vi "Create Device GUI.vi"(8 "Error In":errorcluster, 9 "Device":i32, 10 "Platform":i32, 11 "Skip Configuration":bool) -> (0 "error constant":errorcluster, 3 "Device Reference":T1)   [LabVIEW 2012]
doc: "A GUI that shows which OpenCL Platforms and Devices are available. Selecting a platform will populate the devices available for that platform. Once a device is selected, a context can be created by clicking continue.\n\nThe GUI can be bypassed by wiring <b>Skip Configuration</b> to true and providing a Platform and Device number. This is only recommended after running the GUI and becoming familiar with devices and platforms."
uses:
  Non-User VIs/Controls/Device ID.ctl
  Non-User VIs/Buffers/Buffer_states.ctl
  Non-User VIs/Error Checking/Add Error Functional Global.vi
  OpenCLV x64.lvlib
panel:
  in  "Cancel Button":bool
  in  "Continue":bool caption="Create Device"
  out "Device Properties":string[](tree)
  in  "Devices":i32(listbox)
  out "Platform Properties":string[](tree)=["FULL_PROFILE"]
  in  "Platform Names":i32(listbox)
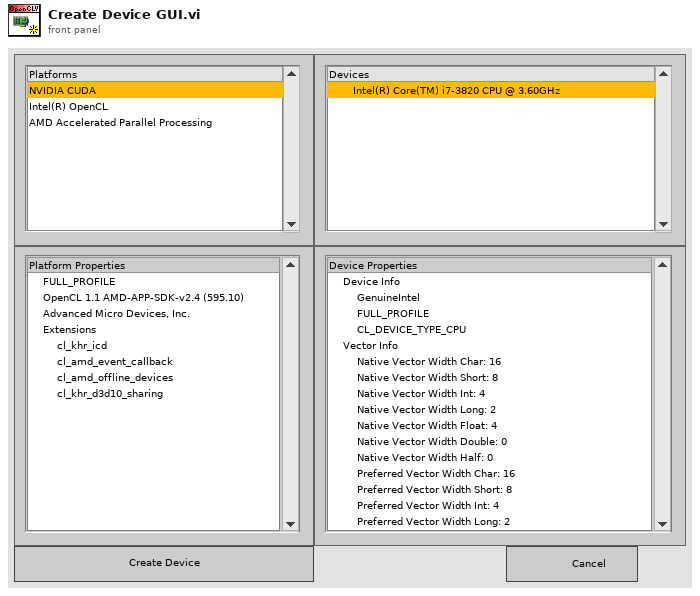
[diagram p1: front panel]
types:
  T1 = typedef "OpenCLV x64.lvlib/Device ID.ctl" = u64
  T2 = typedef "OpenCLV x64.lvlib/Buffer_states.ctl" = enum16{"Purge", "Remove", "Add"}
  T3 = enum8{"Enabled", "Disabled", "Disabled and Grayed Out"}
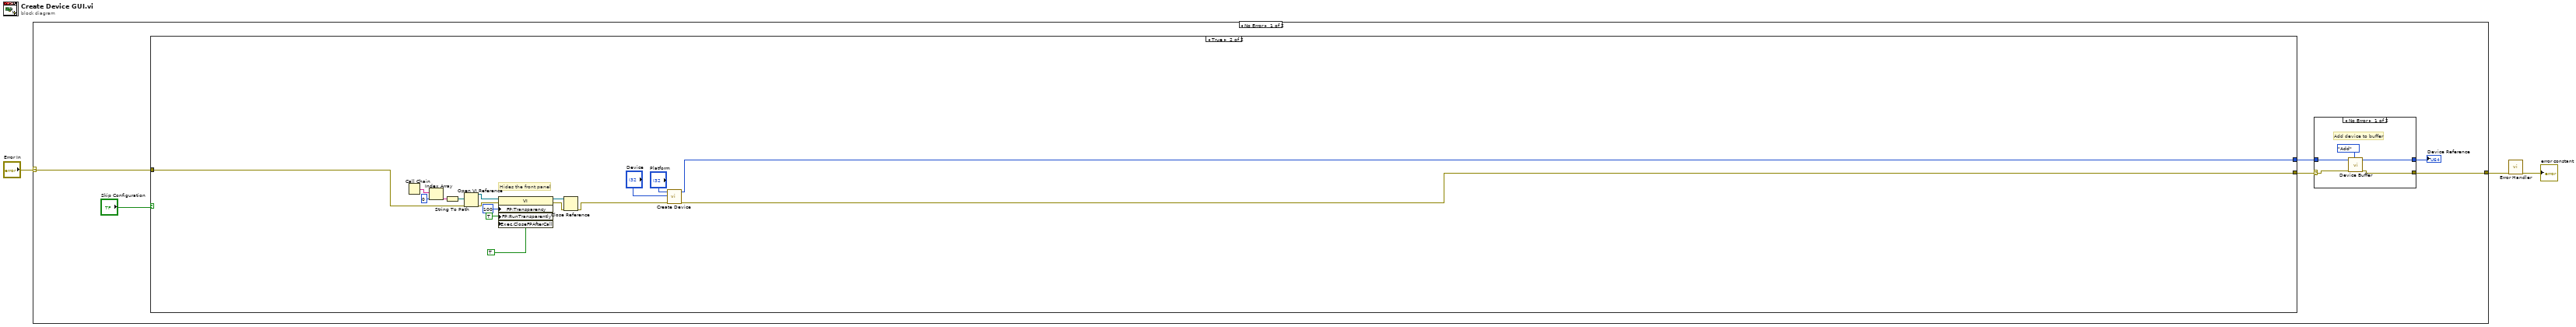
[diagram p0: block diagram]
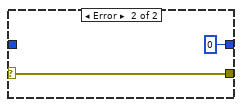
[diagram p2: hidden frame]
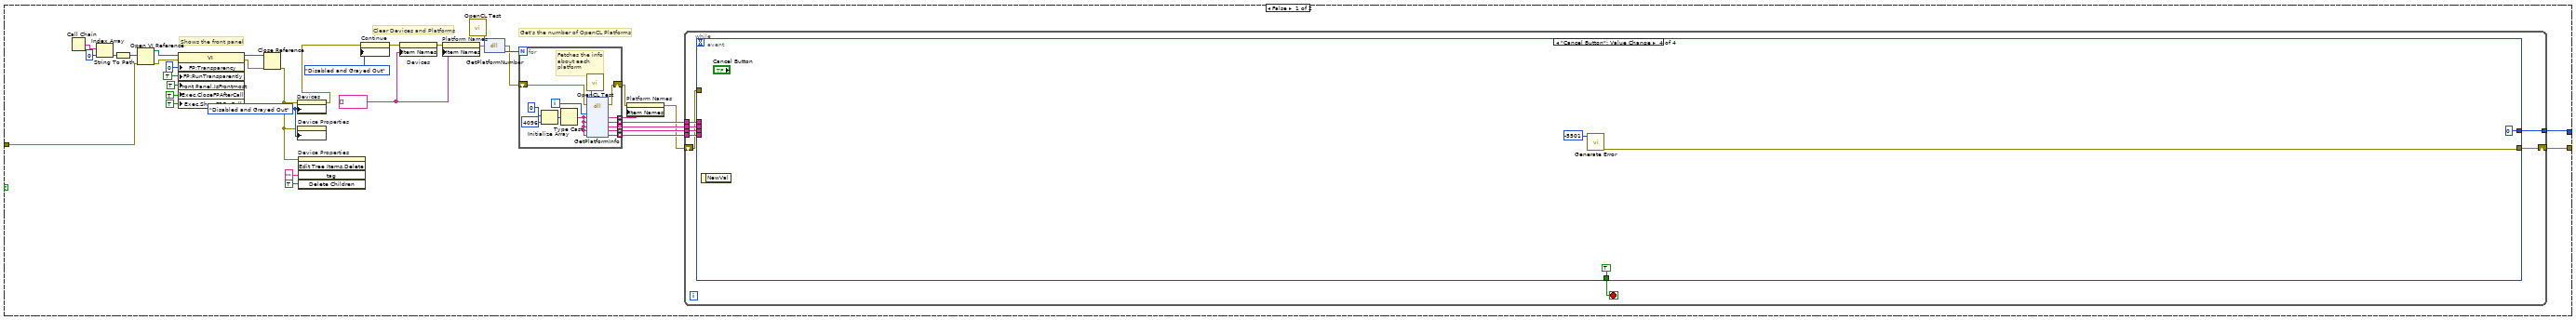
[diagram p3: hidden frame]
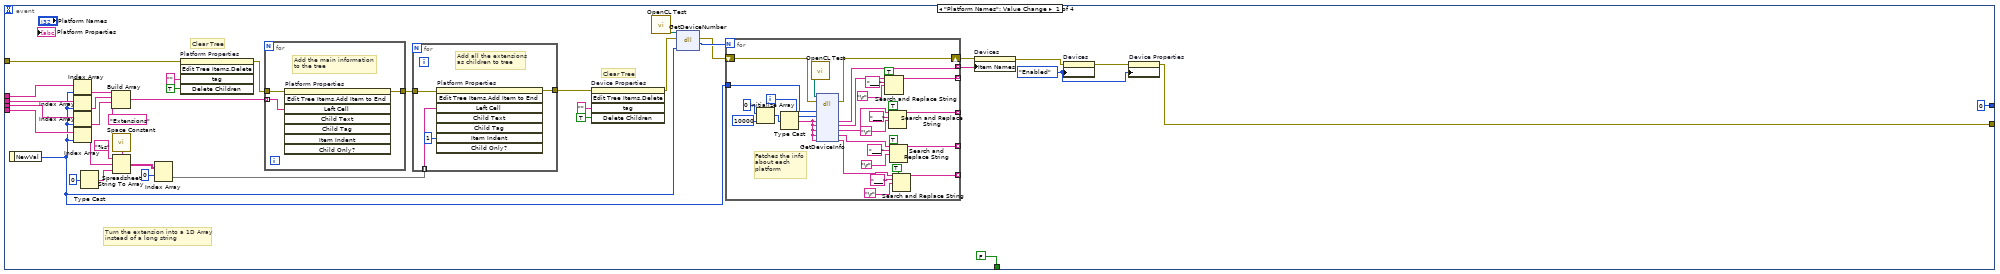
[diagram p4: hidden frame]
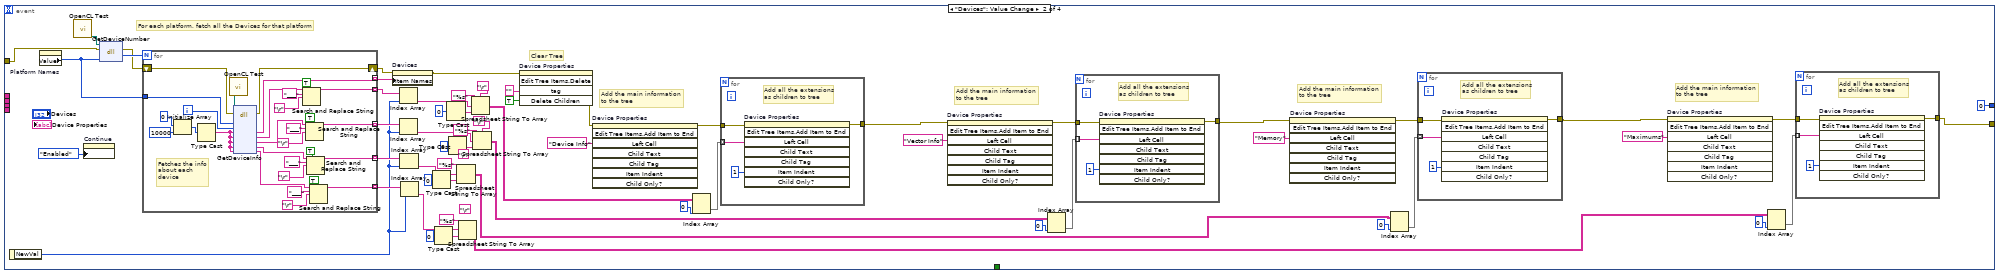
[diagram p5: hidden frame]
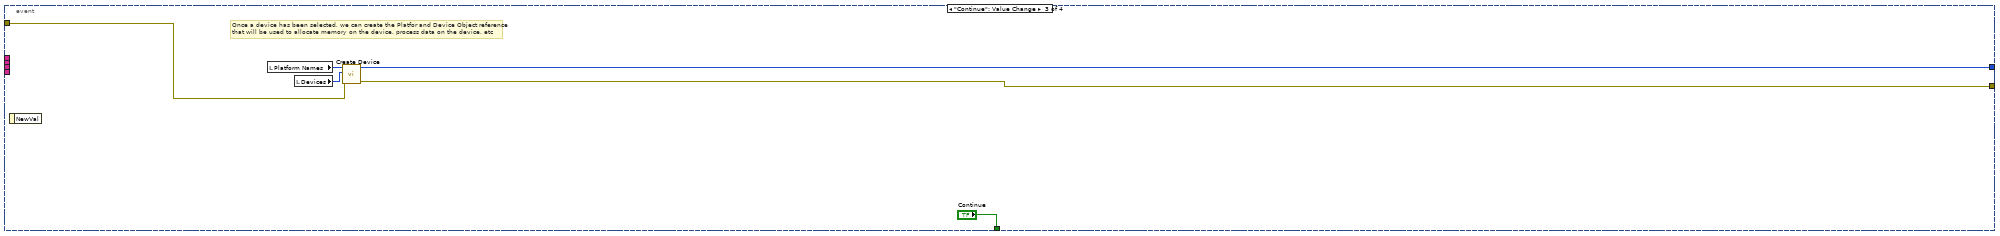
[diagram p6: hidden frame]
diagram:
  n1 = case shown="No Error" "Error In" {
    selector: "Error In" -> [w4 w282]
    tunnel: [w5 w282] -> w2
    frame No Error {
      n2 = case shown="True" "Skip Configuration" {
        tunnel: [w20 w280] -> w7
        tunnel: [w29 w269] -> w8
        tunnel: w4 -> [w17 w265]
        frame False {
          w25 = T3."Disabled and Grayed Out" ("Disabled")
          w43 = string[] [] ("Item Names")
          # "Shows the front panel"
          # "Clear Devices and Platforms"
          # "Get's the number of OpenCL Platforms"
          n3 = Call Chain() -> (call chain=w40:string[])
          n4 = Index Array(array=w40, index=0) -> (element=w38:string)
          n5 = String To Path(string=w38) -> (path=w37:path)
          n6 = Open VI Reference(vi path=w37, error in (no error)=w17) -> (vi reference=w36:refnum<vi>, error out=w35:errorcluster)  [unwired: 4 in]
          n7 = property class="VI"(reference=w36, error in=w35, "FP:Transparency"=u8 0 ("Front Panel Window:Transparency"), "FP:RunTransparently"=TRUE ("Front Panel Window:Run VI Transparently"), "Front Panel.IsFrontmost"=TRUE ("Front Panel Window:Is Frontmost"), "Exec.CloseFPAfterCall"=TRUE ("Execution:Close After Call"), "Exec.ShowFPOnCall"=TRUE ("Execution:Show Front Panel On Call")) -> (reference out=w28:refnum<vi>, error out=w27:errorcluster)
          n8 = Close Reference(reference=w28, error in (no error)=w27) -> (error out=w22:errorcluster)
          n9 = property on="Devices" class="LstBox (strict)"(error in=w22, "DisabledEnum"=w25) -> (error out=w26:errorcluster)  [unwired: 1 in, 1 out]
          n10 = property on="Device Properties" class="Tree (strict)"(error in=w22, "DisabledEnum"=w25) -> ()  [unwired: 1 in, 2 out]
          n11 = invoke on="Device Properties" class="Tree (strict)" method="Edit Tree Items.Delete"(error in=w22, "tag"="" ("Tag"), "Delete Children"=TRUE ("Delete Children?")) -> ()  [unwired: 2 in, 5 out]
          n12 = property on="Continue" class="Bool"(error in=w26, "DisabledEnum"=T3."Disabled and Grayed Out" ("Disabled")) -> (error out=w41:errorcluster)  [unwired: 1 in, 1 out]
          n13 = property on="Devices" class="LstBox (strict)"(error in=w41, "Item Names"=w43) -> (error out=w44:errorcluster)  [unwired: 1 in, 1 out]
          n14 = property on="Platform Names" class="LstBox (strict)"(error in=w44, "Item Names"=w43) -> (error out=w45:errorcluster)  [unwired: 1 in, 1 out]
          n15 = call "OpenCL Test.vi"() -> ("DLL To Use"=w21:path)  [unwired: 11 in]
          n16 = dll-call lib="C:/Users/bme-amcelroy-la/Desktop/OpenCLV/trunk/OpenCLV_x64_1.0/OpenCLV_x64.dll" fn="GetPlatformNumber"(path in=w21, error in=w45) -> (error out=w19:errorcluster, "Number of Platforms"=w47:i32)  [unwired: 1 in, 1 out]
          n17 = for {
            N: w47 -> [_]
            tunnel: [w264] -> w52 mode=indexing
            tunnel: [w262] -> w51 mode=indexing
            tunnel: [w261] -> w50 mode=indexing
            tunnel: [w260] -> w49 mode=indexing
            tunnel: [w259] -> w48 mode=indexing
            shift-right: [w252] -> w18
            shift-left: w19 -> [w253]
            i -> [w263]
            # "Fetches the info\nabout each \nplatform"
            n18 = Initialize Array(u8 0, 4096 ("dimension size")) -> (w256:u8[])
            n19 = Type Cast(x=w256) -> (*(type *) &x=w255:string)  [unwired: 1 in]
            n20 = call "OpenCL Test.vi"() -> ("DLL To Use"=w254:path)  [unwired: 11 in]
            n21 = dll-call lib="C:/Users/bme-amcelroy-la/Desktop/OpenCLV/trunk/OpenCLV_x64_1.0/OpenCLV_x64.dll" fn="GetPlatformInfo"(path in=w254, error in=w253, "Platform ID"=w263, "PlatformNames"=w255, "Platform Profile"=w255, "Platform Version"=w255, "Platform Vendor"=w255, "Platform Extensions"=w255) -> (error out=w252:errorcluster, "PlatformNames"=w264:string, "Platform Profile"=w262:string, "Platform Version"=w261:string, "Platform Vendor"=w260:string, "Platform Extensions"=w259:string)  [unwired: 3 in, 1 out]
          }
          n22 = property on="Platform Names" class="LstBox (strict)"(error in=w18, "Item Names"=w52) -> (error out=w46:errorcluster)  [unwired: 1 in, 1 out]
          n23 = while {
            tunnel: w51 -> [w60]
            tunnel: w50 -> [w59]
            tunnel: w49 -> [w58]
            tunnel: w48 -> [w57]
            tunnel: [w55] -> w29
            shift-right: [w53] -> w20
            shift-left: w46 -> [w54]
            stop <- w56 stop-if-true
            n24 = event shown="[3] \"Cancel Button\": Value Change" {
              selector: _ -> [_ _ _ _]
              dyn-events: _ -> [_ _ _ _]
              timeout: _ -> [_ _ _ _]
              tunnel: w60 -> [w78 _ _ _]
              tunnel: w59 -> [w97 _ _ _]
              tunnel: w58 -> [w98 _ _ _]
              tunnel: w57 -> [w91 _ _ _]
              tunnel: [FALSE _ "Continue" TRUE ("Continue")] -> w56
              tunnel: [w64 w137 w244 w250] -> w53
              tunnel: [T1 0 ("Device Reference") T1 0 ("Device Reference") w243 T1 0 ("Device Reference")] -> w55
              tunnel: w54 -> [w66 w140 w242 _]
              event "Platform Names": Value Change {
                w68 = T3."Enabled" ("Disabled")
                # "Clear Tree"
                # "Turn the extension into a 1D Array\ninstead of a long string"
                # "Clear Tree"
                n25 = event-data() -> ("NewVal"=w71:i32)  [unwired: 1 in]
                n26 = Index Array(array=w78, index=w71) -> (element=w96:string)
                n27 = Index Array(array=w97, index=w71) -> (element=w95:string)
                n28 = Index Array(array=w98, index=w71) -> (element=w94:string)
                n29 = Index Array(array=w91, index=w71) -> (element=w85:string)
                n30 = Type Cast(x=u8 0) -> (*(type *) &x=w84:string)  [unwired: 1 in]
                n31 = Build Array(w96, w95, w94, "Extensions" ("element")) -> (w92:string[])
                n32 = call <vilib>:"Space Constant.vi"() -> ("String"=w87:string)
                n33 = Spreadsheet String To Array(delimiter (Tab)=w87, format string="%s", spreadsheet string=w85, array type (2D Dbl)=w84) -> (array=w81:string[][])
                n34 = Index Array(array=w81, index (row)=0) -> (element=w79:string[])  [unwired: 1 in]
                n35 = invoke on="Platform Properties" class="Tree (strict)" method="Edit Tree Items.Delete"(error in=w66, "tag"="" ("Tag"), "Delete Children"=TRUE ("Delete Children?")) -> (error out=w88:errorcluster)  [unwired: 2 in, 4 out]
                n36 = for {
                  tunnel: w92 -> [w135] mode=indexing
                  tunnel: w88 -> [w134]
                  tunnel: [w133] -> w83
                  # "Add the main information\nto the tree"
                  n37 = invoke on="Platform Properties" class="Tree (strict)" method="Edit Tree Items.Add Item to End"(error in=w134, "Left Cell"=w135) -> (error out=w133:errorcluster)  [unwired: 6 in, 7 out]
                }
                n38 = for {
                  tunnel: w83 -> [w132]
                  tunnel: w79 -> [w131] mode=indexing
                  tunnel: [w129] -> w74
                  # "Add all the extensions\nas children to tree"
                  n39 = invoke on="Platform Properties" class="Tree (strict)" method="Edit Tree Items.Add Item to End"(error in=w132, "Left Cell"=w131, "Item Indent"=1 ("New Item Indentation")) -> (error out=w129:errorcluster)  [unwired: 5 in, 7 out]
                }
                n40 = invoke on="Device Properties" class="Tree (strict)" method="Edit Tree Items.Delete"(error in=w74, "tag"="" ("Tag"), "Delete Children"=TRUE ("Delete Children?")) -> (error out=w70:errorcluster)  [unwired: 2 in, 4 out]
                n41 = call "OpenCL Test.vi"() -> ("DLL To Use"=w67:path)  [unwired: 11 in]
                n42 = dll-call lib="C:/Users/bme-amcelroy-la/Desktop/OpenCLV/trunk/OpenCLV_x64_1.0/OpenCLV_x64.dll" fn="GetDeviceNumber"(path in=w67, error in=w70, "Platform"=w71) -> (error out=w63:errorcluster, "Number of Platforms"=w72:i32)  [unwired: 2 in, 1 out]
                n43 = for {
                  N: w72 -> [_]
                  tunnel: w71 -> [w125]
                  tunnel: [w122] -> w73 mode=indexing
                  tunnel: [w105] -> _ mode=indexing
                  tunnel: [w104] -> _ mode=indexing
                  tunnel: [w103] -> _ mode=indexing
                  tunnel: [w102] -> _ mode=indexing
                  shift-right: [w99] -> w62
                  shift-left: w63 -> [w100]
                  i -> [w126]
                  # "Fetches the info\nabout each \nplatform"
                  n44 = Initialize Array(u8 0, 10000 ("dimension size")) -> (w124:u8[])
                  n45 = Type Cast(x=w124) -> (*(type *) &x=w123:string)  [unwired: 1 in]
                  n46 = call "OpenCL Test.vi"() -> ("DLL To Use"=w101:path)  [unwired: 11 in]
                  n47 = dll-call lib="C:/Users/bme-amcelroy-la/Desktop/OpenCLV/trunk/OpenCLV_x64_1.0/OpenCLV_x64.dll" fn="GetDeviceInfo"(path in=w101, error in=w100, "Platform ID"=w125, "Device ID"=w126, "Device Name"=w123, "Device Info"=w123, "Vector Info"=w123, "Memory"=w123, "Maximums"=w123) -> (error out=w99:errorcluster, "Device Name"=w122:string, "Device Info"=w121:string, "Vector Info"=w109:string, "Memory"=w108:string, "Maximums"=w106:string)  [unwired: 4 in, 1 out]
                  n48 = Search and Replace String(replace all?=TRUE ("replace all? (F)"), input string=w121, search string="___", replace string="\r") -> (result string=w105:string)  [unwired: 4 in, 3 out]
                  n49 = Search and Replace String(replace all?=TRUE ("replace all? (F)"), input string=w109, search string="___", replace string="\r") -> (result string=w104:string)  [unwired: 4 in, 3 out]
                  n50 = Search and Replace String(replace all?=TRUE ("replace all? (F)"), input string=w108, search string="___", replace string="\r") -> (result string=w103:string)  [unwired: 4 in, 3 out]
                  n51 = Search and Replace String(replace all?=TRUE ("replace all? (F)"), input string=w106, search string="___", replace string="\r") -> (result string=w102:string)  [unwired: 4 in, 3 out]
                }
                n52 = property on="Devices" class="LstBox (strict)"(error in=w62, "Item Names"=w73) -> (error out=w69:errorcluster)  [unwired: 1 in, 1 out]
                n53 = property on="Devices" class="LstBox (strict)"(error in=w69, "DisabledEnum"=w68) -> (error out=w65:errorcluster)  [unwired: 1 in, 1 out]
                n54 = property on="Device Properties" class="Tree (strict)"(error in=w65, "DisabledEnum"=w68) -> (error out=w64:errorcluster)  [unwired: 1 in, 1 out]
              }
              event "Devices": Value Change {
                (unwired) "\r"
                (unwired) "\r"
                # "Add the main information\nto the tree"
                # "Add the main information\nto the tree"
                # "Add the main information\nto the tree"
                # "Add the main information\nto the tree"
                # "Clear Tree"
                # "For each platform, fetch all the Devices for that platform"
                n55 = event-data() -> ("NewVal"=w143:i32)  [unwired: 1 in]
                n56 = property on="Platform Names" class="LstBox (strict)"() -> ("Value"=w193:i32)  [unwired: 2 in, 2 out]
                n57 = call "OpenCL Test.vi"() -> ("DLL To Use"=w142:path)  [unwired: 11 in]
                n58 = property on="Continue" class="Bool"("DisabledEnum"=T3."Enabled" ("Disabled")) -> ()  [unwired: 2 in, 2 out]
                n59 = dll-call lib="C:/Users/bme-amcelroy-la/Desktop/OpenCLV/trunk/OpenCLV_x64_1.0/OpenCLV_x64.dll" fn="GetDeviceNumber"(path in=w142, error in=w140, "Platform"=w193) -> (error out=w139:errorcluster, "Number of Platforms"=w195:i32)  [unwired: 2 in, 1 out]
                n60 = for {
                  N: w195 -> [_]
                  tunnel: w193 -> [w238]
                  tunnel: [w235] -> w194 mode=indexing
                  tunnel: [w218] -> w192 mode=indexing
                  tunnel: [w217] -> w191 mode=indexing
                  tunnel: [w216] -> w190 mode=indexing
                  tunnel: [w215] -> w189 mode=indexing
                  shift-right: [w212] -> w138
                  shift-left: w139 -> [w213]
                  i -> [w239]
                  # "Fetches the info\nabout each \ndevice"
                  n61 = Initialize Array(u8 0, 10000 ("dimension size")) -> (w237:u8[])
                  n62 = Type Cast(x=w237) -> (*(type *) &x=w236:string)  [unwired: 1 in]
                  n63 = call "OpenCL Test.vi"() -> ("DLL To Use"=w214:path)  [unwired: 11 in]
                  n64 = dll-call lib="C:/Users/bme-amcelroy-la/Desktop/OpenCLV/trunk/OpenCLV_x64_1.0/OpenCLV_x64.dll" fn="GetDeviceInfo"(path in=w214, error in=w213, "Platform ID"=w238, "Device ID"=w239, "Device Name"=w236, "Device Info"=w236, "Vector Info"=w236, "Memory"=w236, "Maximums"=w236) -> (error out=w212:errorcluster, "Device Name"=w235:string, "Device Info"=w234:string, "Vector Info"=w222:string, "Memory"=w221:string, "Maximums"=w219:string)  [unwired: 4 in, 1 out]
                  n65 = Search and Replace String(replace all?=TRUE ("replace all? (F)"), input string=w234, search string="___", replace string="\r") -> (result string=w218:string)  [unwired: 4 in, 3 out]
                  n66 = Search and Replace String(replace all?=TRUE ("replace all? (F)"), input string=w222, search string="___", replace string="\r") -> (result string=w217:string)  [unwired: 4 in, 3 out]
                  n67 = Search and Replace String(replace all?=TRUE ("replace all? (F)"), input string=w221, search string="___", replace string="\r") -> (result string=w216:string)  [unwired: 4 in, 3 out]
                  n68 = Search and Replace String(replace all?=TRUE ("replace all? (F)"), input string=w219, search string="___", replace string="\r") -> (result string=w215:string)  [unwired: 4 in, 3 out]
                }
                n69 = property on="Devices" class="LstBox (strict)"(error in=w138, "Item Names"=w194) -> (error out=w186:errorcluster)  [unwired: 1 in, 1 out]
                n70 = Index Array(array=w192, index=w143) -> (element=w180:string)
                n71 = Index Array(array=w191, index=w143) -> (element=w167:string)
                n72 = Index Array(array=w190, index=w143) -> (element=w152:string)
                n73 = Index Array(array=w189, index=w143) -> (element=w151:string)
                n74 = Type Cast(x=u8 0) -> (*(type *) &x=w157:string)  [unwired: 1 in]
                n75 = Type Cast(x=u8 0) -> (*(type *) &x=w154:string)  [unwired: 1 in]
                n76 = Type Cast(x=u8 0) -> (*(type *) &x=w181:string)  [unwired: 1 in]
                n77 = Type Cast(x=u8 0) -> (*(type *) &x=w168:string)  [unwired: 1 in]
                n78 = Spreadsheet String To Array(format string="%s", spreadsheet string=w152, array type (2D Dbl)=w157) -> (array=w150:string[][])  [unwired: 1 in]
                n79 = Spreadsheet String To Array(format string="%s", spreadsheet string=w151, array type (2D Dbl)=w154) -> (array=w144:string[][])  [unwired: 1 in]
                n80 = Spreadsheet String To Array(delimiter (Tab)="\r", format string="%s", spreadsheet string=w180, array type (2D Dbl)=w181) -> (array=w177:string[][])
                n81 = Spreadsheet String To Array(delimiter (Tab)="\r", format string="%s", spreadsheet string=w167, array type (2D Dbl)=w168) -> (array=w164:string[][])
                n82 = invoke on="Device Properties" class="Tree (strict)" method="Edit Tree Items.Delete"(error in=w186, "tag"="" ("Tag"), "Delete Children"=TRUE ("Delete Children?")) -> (error out=w184:errorcluster)  [unwired: 2 in, 4 out]
                n83 = invoke on="Device Properties" class="Tree (strict)" method="Edit Tree Items.Add Item to End"(error in=w184, "Left Cell"="Device Info" ("Left Cell String")) -> (error out=w185:errorcluster)  [unwired: 6 in, 7 out]
                n84 = Index Array(array=w177, index (col)=0 ("index (row)")) -> (element=w176:string[])  [unwired: 1 in]
                n85 = for {
                  tunnel: w185 -> [w211]
                  tunnel: [w209] -> w170
                  tunnel: w176 -> [w208] mode=indexing
                  # "Add all the extensions\nas children to tree"
                  n86 = invoke on="Device Properties" class="Tree (strict)" method="Edit Tree Items.Add Item to End"(error in=w211, "Left Cell"=w208, "Item Indent"=1 ("New Item Indentation")) -> (error out=w209:errorcluster)  [unwired: 5 in, 7 out]
                }
                n87 = invoke on="Device Properties" class="Tree (strict)" method="Edit Tree Items.Add Item to End"(error in=w170, "Left Cell"="Vector Info" ("Left Cell String")) -> (error out=w171:errorcluster)  [unwired: 6 in, 7 out]
                n88 = Index Array(array=w164, index (col)=0 ("index (row)")) -> (element=w173:string[])  [unwired: 1 in]
                n89 = for {
                  tunnel: w171 -> [w207]
                  tunnel: [w205] -> w159
                  tunnel: w173 -> [w204] mode=indexing
                  # "Add all the extensions\nas children to tree"
                  n90 = invoke on="Device Properties" class="Tree (strict)" method="Edit Tree Items.Add Item to End"(error in=w207, "Left Cell"=w204, "Item Indent"=1 ("New Item Indentation")) -> (error out=w205:errorcluster)  [unwired: 5 in, 7 out]
                }
                n91 = invoke on="Device Properties" class="Tree (strict)" method="Edit Tree Items.Add Item to End"(error in=w159, "Left Cell"="Memory" ("Left Cell String")) -> (error out=w163:errorcluster)  [unwired: 6 in, 7 out]
                n92 = Index Array(array=w150, index (col)=0 ("index (row)")) -> (element=w161:string[])  [unwired: 1 in]
                n93 = for {
                  tunnel: w163 -> [w203]
                  tunnel: [w201] -> w145
                  tunnel: w161 -> [w200] mode=indexing
                  # "Add all the extensions\nas children to tree"
                  n94 = invoke on="Device Properties" class="Tree (strict)" method="Edit Tree Items.Add Item to End"(error in=w203, "Left Cell"=w200, "Item Indent"=1 ("New Item Indentation")) -> (error out=w201:errorcluster)  [unwired: 5 in, 7 out]
                }
                n95 = invoke on="Device Properties" class="Tree (strict)" method="Edit Tree Items.Add Item to End"(error in=w145, "Left Cell"="Maximums" ("Left Cell String")) -> (error out=w146:errorcluster)  [unwired: 6 in, 7 out]
                n96 = Index Array(array=w144, index (col)=0 ("index (row)")) -> (element=w148:string[])  [unwired: 1 in]
                n97 = for {
                  tunnel: w146 -> [w199]
                  tunnel: [w197] -> w137
                  tunnel: w148 -> [w196] mode=indexing
                  # "Add all the extensions\nas children to tree"
                  n98 = invoke on="Device Properties" class="Tree (strict)" method="Edit Tree Items.Add Item to End"(error in=w199, "Left Cell"=w196, "Item Indent"=1 ("New Item Indentation")) -> (error out=w197:errorcluster)  [unwired: 5 in, 7 out]
                }
              }
              event "Continue": Value Change {
                # "Once a device has been selected, we can create the Platfor and Device Object reference\nthat will be used to allocate memory on the device, process data on the device, etc"
                n99 = event-data() -> ()  [unwired: 1 in, 1 out]
                n100 = local read "Platform Names"() -> (w246:i32)
                n101 = local read "Devices"() -> (w245:i32)
                n102 = call "Create Device.vi"("Error In"=w242, "Devices"=w245, "Platform Names"=w246) -> ("error out"=w244:errorcluster, "Device Reference"=w243:T1)  [unwired: 7 in]
              }
              event "Cancel Button": Value Change {
                n103 = event-data() -> ()  [unwired: 1 in, 1 out]
                n104 = call "Generate Error.vi"("Error"=-5501) -> ("error out"=w250:errorcluster)  [unwired: 10 in]
              }
            }
          }
        }
        frame True {
          # "Hides the front panel"
          n105 = Call Chain() -> (call chain=w279:string[])
          n106 = Index Array(array=w279, index=0) -> (element=w277:string)
          n107 = String To Path(string=w277) -> (path=w276:path)
          n108 = Open VI Reference(vi path=w276, error in (no error)=w265) -> (vi reference=w275:refnum<vi>, error out=w274:errorcluster)  [unwired: 4 in]
          n109 = property class="VI"(reference=w275, error in=w274, "FP:Transparency"=u8 100 ("Front Panel Window:Transparency"), "FP:RunTransparently"=TRUE ("Front Panel Window:Run VI Transparently"), "Exec.CloseFPAfterCall"=TRUE ("Execution:Close After Call")) -> (reference out=w268:refnum<vi>, error out=w267:errorcluster)
          n110 = Close Reference(reference=w268, error in (no error)=w267) -> (error out=w266:errorcluster)
          n111 = call "Create Device.vi"("Error In"=w266, "Devices"="Device", "Platform Names"="Platform") -> ("error out"=w280:errorcluster, "Device Reference"=w269:T1)  [unwired: 7 in]
        }
      }
      n112 = case shown="No Error" w7 {
        selector: w7 -> [w11 w16]
        tunnel: [w14 w16] -> w5
        tunnel: w8 -> [w13 _]
        tunnel: [w10 T1 0 ("Device Out")] -> w6
        frame No Error {
          # "Add device to buffer"
          n113 = call "Device Buffer.vi"("States"=Buffer_states."Add", "Error In"=w11, "Device"=w13) -> ("Error Out"=w14:errorcluster, "Device Out"=w10:T1)  [unwired: 7 in]
        }
        frame Error {
        }
      }
      "Device Reference" <- w6
    }
    frame Error {
    }
  }
  n114 = call-poly "Error Handler.vi"("Error In"=w2) -> ("Error Out"=→"error constant":errorcluster)  [unwired: 10 in]
